vi "Test0823.vi"() -> ()   [LabVIEW 2016]
uses:
  LV-EDSDK-Distribution_0.2/Distribution/EDSDK-Labview.llb/EdsImageInfo.ctl
  LV-EDSDK-Distribution_0.2/Distribution/EDSDK-Labview.llb/kEdsProperties.ctl
  LV-EDSDK-Distribution_0.2/Distribution/EDSDK-Labview.llb/kEdsImageSrcs.ctl
  EDSDK131020CD(13.10.20)/EDSDK131020CD(13.10.20)/Windows/EDSDK_64/Dll/EDSDK.dll
  Dll for liveview/x64/Debug/Dll for liveview.dll
panel:
  out "2D Picture":picture
  out "Intensity Graph":u32[][](graph)
  out "output array":u32[][](array[numeric])
  out "return type 3":i32
  out "return type 2":i32
  in  "EdsRect":T1
  in  "EdsSize":cluster{"height":i32, "width":i32}
  out "return type":i32
  out "inStreamRef dup":i32
  out "outImageInfo":T2
  out "outDeviceInfo":T3
  out "error out":errorcluster
  in  "error in (no error)":errorcluster
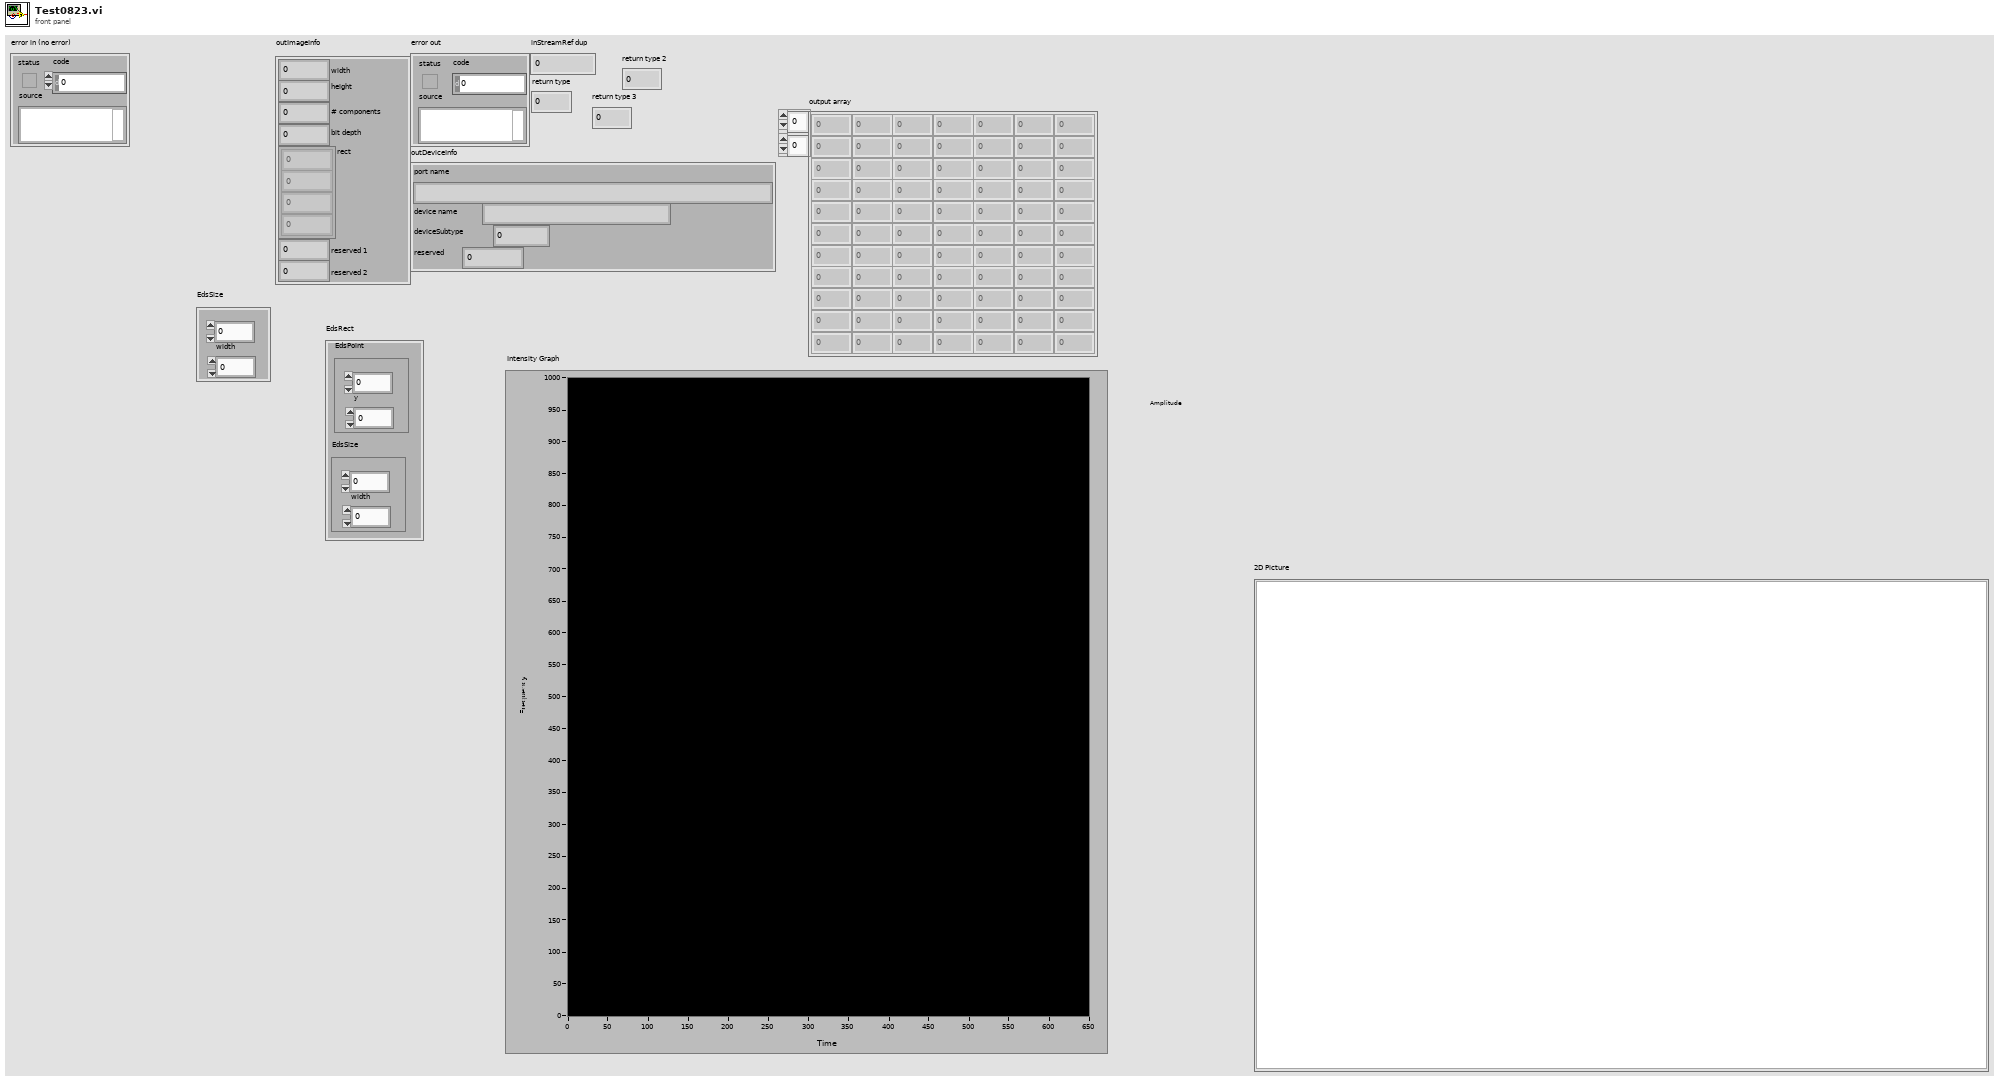
[diagram p1: front panel]
types:
  T1 = cluster{"EdsPoint":cluster{"x":i32, "y":i32}, "EdsSize":cluster{"height":i32, "width":i32}}
  T2 = typedef "EdsImageInfo.ctl" = cluster{"width":u32, "height":u32, "# components":u32, "bit depth":u32, "rect":u32[], "reserved 1":u32, "reserved 2":u32}
  T3 = cluster{"port name":string, "device name":string, "deviceSubtype":u32, "reserved":u32}
  T4 = typedef "kEdsProperties.ctl" = u32
  T5 = typedef "kEdsImageSrcs.ctl" = u32
  T6 = typedef "imagedata.ctl" = cluster{"image type":i32, "image depth":i32, "image":u8[], "mask":u8[], "colors":u32[], "Rectangle":cluster{"left":i16, "top":i16, "right":i16, "bottom":i16}}
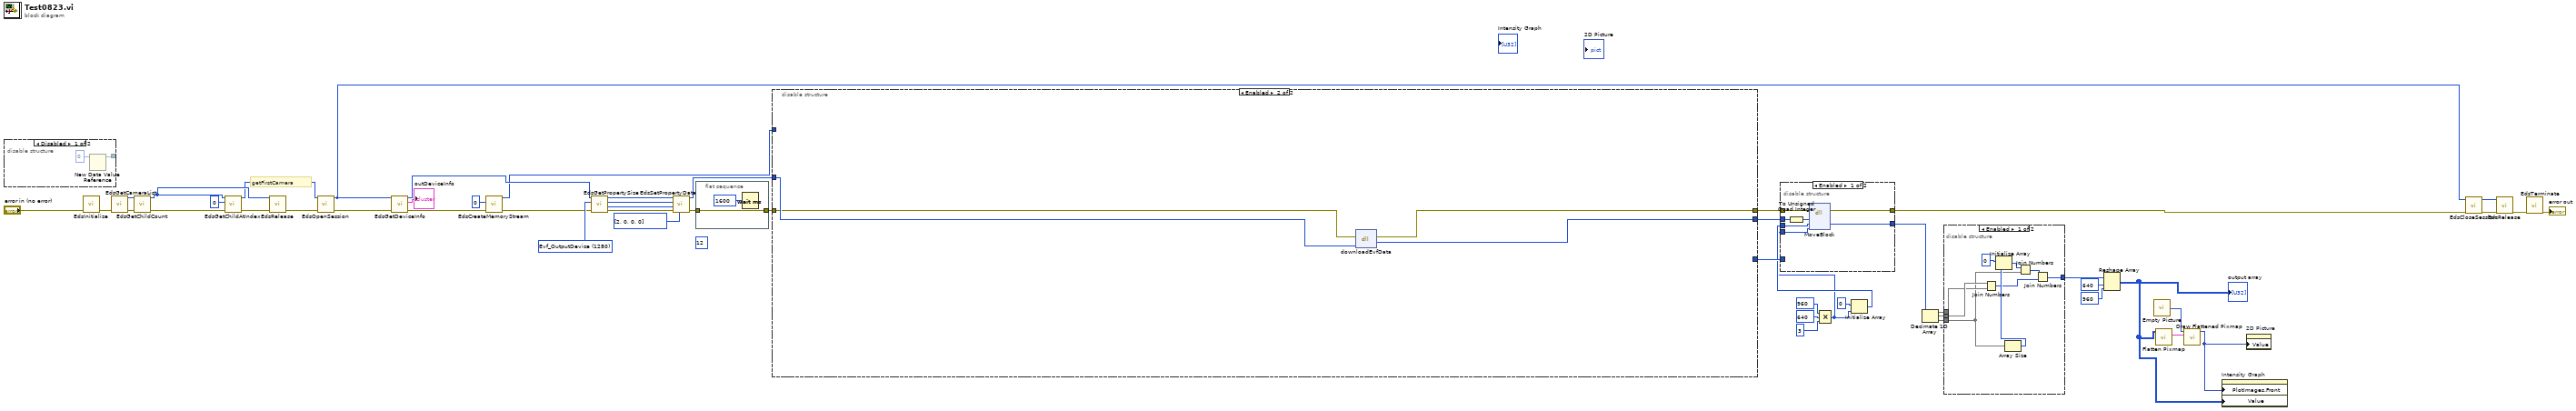
[diagram p0: block diagram]
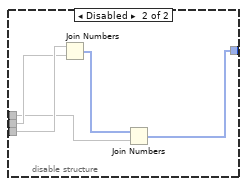
[diagram p2: hidden frame]
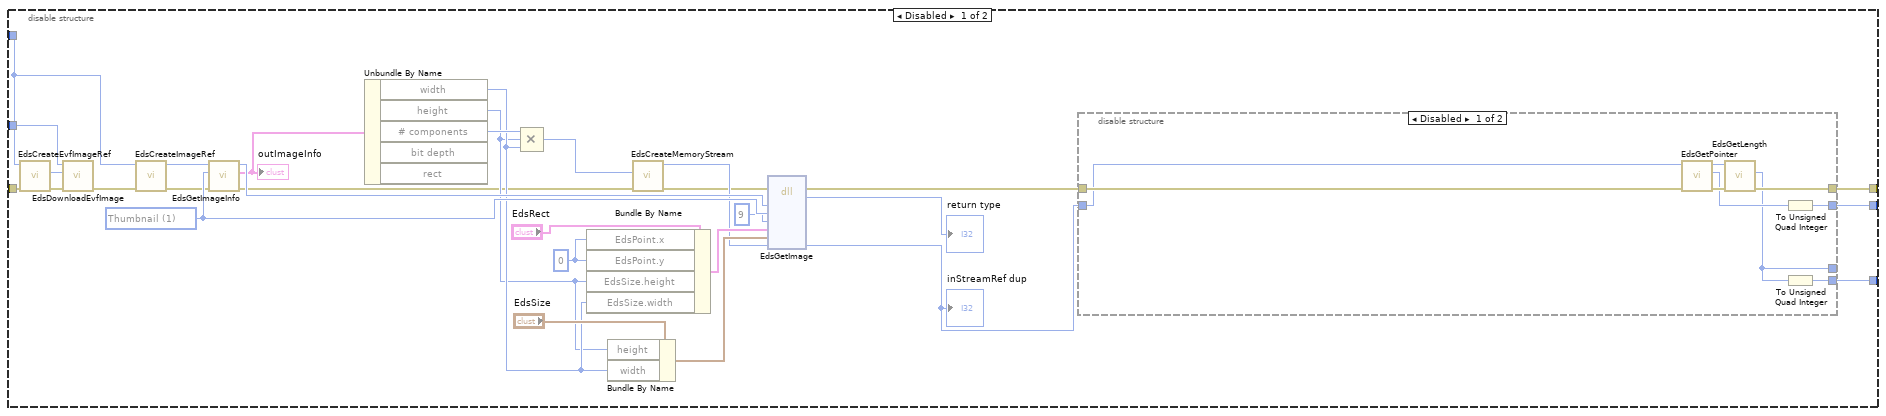
[diagram p3: hidden frame]
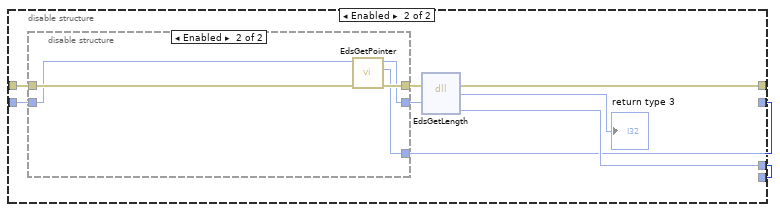
[diagram p4: hidden frame]
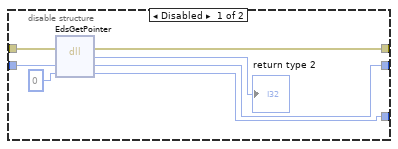
[diagram p5: hidden frame]
diagram:
  (unwired) u8 12 ("element")
  w36 = T4 1280 items=["Unknown"=65535, "ProductName"=2, "BodyID"=3, "OwnerName"=4, "MakerName"=5, "DateTime"=6, "FirmwareVersion"=7, "BatteryLevel"=8, "CFn"=9, "SaveTo"=11, "CurrentStorage"=12, "CurrentFolder"=13, "MyMenu"=14, "BatteryQuality"=16, "HDDirectoryStructure"=32, "ImageQuality"=256, "JpegQuality"=257, "Orientation"=258, "ICCProfile"=259, "FocusInfo"=260, "DigitalExposure"=261, "WhiteBalance"=262, "ColorTemperature"=263, "WhiteBalanceShift"=264, "Contrast"=265, "ColorSaturation"=266, "ColorTone"=267, "Sharpness"=268, "ColorSpace"=269, "ToneCurve"=270, "PhotoEffect"=271, "FilterEffect"=272, "ToningEffect"=273, "ParameterSet"=274, "ColorMatrix"=275, "PictureStyle"=276, "PictureStyleDesc"=277, "ETTL2Mode"=279, "PictureStyleCaption"=512, "Linear"=768, "ClickWBPoint"=769, "WBCoeffs"=770, "GPSVersionID"=2048, "GPSLatitudeRef"=2049, "GPSLatitude"=2050, "GPSLongitudeRef"=2051, "GPSLongitude"=2052, "GPSAltitudeRef"=2053, "GPSAltitude"=2054, "GPSTimeStamp"=2055, "GPSSatellites"=2056, "GPSStatus"=2057, "GPSMapDatum"=2066, "GPSDateStamp"=2077, "AtCapture_Flag"=2147483648, "AEMode"=1024, "DriveMode"=1025, "ISOSpeed"=1026, "MeteringMode"=1027, "AFMode"=1028, "Av"=1029, "Tv"=1030, "ExposureCompensation"=1031, "FlashCompensation"=1032, "FocalLength"=1033, "AvailableShots"=1034, "Bracket"=1035, "WhiteBalanceBracket"=1036, "LensName"=1037, "AEBracket"=1038, "FEBracket"=1039, "ISOBracket"=1040, "NoiseReduction"=1041, "FlashOn"=1042, "RedEye"=1043, "FlashMode"=1044, "LensStatus"=1046, "Artist"=1048, "Copyright"=1049, "DepthOfField"=1051, "EFCompensation"=1054, "Evf_OutputDevice"=1280, "Evf_Mode"=1281, "Evf_WhiteBalance"=1282, "Evf_ColorTemperature"=1283, "Evf_DepthOfFieldPreview"=1284, "Evf_Zoom"=1287, "Evf_ZoomPosition"=1288, "Evf_FocusAid"=1289, "Evf_Histogram"=1290, "Evf_ImagePosition"=1291, "Evf_HistogramStatus"=1292, "Evf_AFMode"=1294, "Evf_CoordinateSystem"=1344, "Evf_ZoomRect"=1345] ("inPropertyID")
  # "getFirstCamera"
  n1 = disable-structure shown="Disabled" {
    disable-tunnel: [w53 _] -> _
    frame Disabled {
      n2 = New Data Value Reference(data value=i64 0) -> (data value reference=w53:refnum<data-value>)  [unwired: 1 in, 1 out]
    }
    frame Enabled {
    }
  }
  n3 = call "EdsInitialize.vi"("error in (no error)"="error in (no error)") -> ("error out"=w51:errorcluster)  [unwired: 10 in]
  n4 = call "EdsGetCameraList.vi"("error in"=w51) -> ("error out"=w50:errorcluster, "outCameraListRef"=w46:u32)  [unwired: 9 in]
  n5 = call "EdsGetChildCount.vi"("error in"=w50, "inRef"=w46) -> ("error out"=w49:errorcluster, "inRef dup"=w45:u32)  [unwired: 7 in, 1 out]
  n6 = call "EdsGetChildAtIndex.vi"("error in"=w49, "index"=u32 0, "inRef"=w45) -> ("error out"=w47:errorcluster, "outRef"=w40:u32)  [unwired: 7 in]
  n7 = call "EdsRelease.vi"("error in"=w47, "inRef"=w45) -> ("error out"=w44:errorcluster)  [unwired: 7 in, 2 out]
  n8 = call "EdsOpenSession.vi"("error in"=w44, "inCameraRef"=w40) -> ("error out"=w38:errorcluster, "inCameraRef dup"=w39:u32)  [unwired: 8 in]
  n9 = call "EdsGetDeviceInfo.vi"("error in"=w38, "inCameraRef"=w39) -> ("error out"=w28:errorcluster, "outDeviceInfo"=→"outDeviceInfo":T3, "inCameraRef dup"=w29:u32)  [unwired: 7 in]
  n10 = call "EdsCreateMemoryStream.vi"("error in"=w28, "inBufferSize"=u32 0) -> ("error out"=w30:errorcluster, "outStreamRef"=w23:u32)  [unwired: 8 in]
  n11 = call "EdsGetPropertySize.vi"("error in"=w30, "inPropertyID"=w36, "inRef"=w29) -> ("error out"=w33:errorcluster, "outSize"=w32:u32, "inPropertyID dup"=w34:T4, "inRef dup"=w35:u32)  [unwired: 4 in, 1 out]
  n12 = call "EdsSetPropertyData.vi"("inPropertyData"=u8[] [2, 0, 0, 0], "error in"=w33, "inPropertySize"=w32, "inPropertyID"=w34, "inRef"=w35) -> ("error out"=w21:errorcluster, "inRef dup"=w26:u32)  [unwired: 5 in]
  n13 = flat-sequence {
    tunnel: w21 -> [w56]
    tunnel: [w56] -> w20
    frame #0 {
      n14 = Wait (ms)(milliseconds to wait=u32 1600) -> ()  [unwired: 1 out]
    }
  }
  n15 = disable-structure shown="Enabled" {
    disable-tunnel: w26 -> [w84 w119]
    disable-tunnel: [w72 _] -> w24
    disable-tunnel: w23 -> [w63 _]
    disable-tunnel: [w62 w117] -> w22
    disable-tunnel: w20 -> [w61 w118]
    disable-tunnel: [w60 w116] -> w6
    frame Disabled {
      w76 = 0 ("x")
      w81 = T5 1 items=["FullView", "Thumbnail", "Preview", "RAWThumbnail", "RAWFullView"] ("inImageSource")
      n16 = call "EdsCreateEvfImageRef.vi"("error in"=w61, "inStream"=w63) -> ("error out"=w86:errorcluster, "outEvfImage"=w85:u32)  [unwired: 7 in, 1 out]
      n17 = call "EdsDownloadEvfImage.vi"("error in"=w86, "inEvfImageRef"=w85, "inCameraRef"=w84) -> ("error out"=w66:errorcluster)  [unwired: 6 in, 2 out]
      n18 = call "EdsCreateImageRef.vi"("error in"=w66, "inStreamRef"=w63) -> ("error out"=w65:errorcluster, "outImageRef"=w64:u32)  [unwired: 8 in]
      n19 = call "EdsGetImageInfo.vi"("error in"=w65, "inImageSource"=w81, "inImageRef"=w64) -> ("error out"=w58:errorcluster, "outImageInfo"=w82:T2, "inImageRef dup"=w83:u32)  [unwired: 6 in]
      "outImageInfo" <- w82
      n20 = Unbundle By Name(w82) -> ("width"=w71:u32, "height"=w70:u32, "# components"=w80:u32)  [unwired: 2 out]
      n21 = Compound Arithmetic op=MULTIPLY(w80, w70, w71) -> (w68:u32)
      n22 = Bundle By Name(cluster="EdsRect", "EdsPoint.x"=w76, "EdsPoint.y"=w76, "EdsSize.height"=w70, "EdsSize.width"=w71) -> (w74:T1)
      n23 = Bundle By Name(cluster="EdsSize", "height"=w70, "width"=w71) -> (w73:cluster{"height":i32, "width":i32})
      n24 = call "EdsCreateMemoryStream.vi"("error in"=w58, "inBufferSize"=w68) -> ("error out"=w57:errorcluster, "outStreamRef"=w67:u32)  [unwired: 8 in]
      n25 = dll-call lib="D:/All Users/Summer2019/Camera_po_sheng/Canon/EDSDK131020CD(13.10.20)/EDSDK131020CD(13.10.20)/Windows/EDSDK_64/Dll/EDSDK.dll" fn="EdsGetImage"(error in=w57, "inImageRef"=w83, "inImageSource"=w81, "inImageType"=9, "inSrcRect"=w74, "inDstSize"=w73, "outStreamRef"=w67) -> (error out=w59:errorcluster, "return type"=→"return type":i32, "outStreamRef"=w69:u32)  [unwired: 7 in, 1 out]
      "inStreamRef dup" <- w69
      n26 = disable-structure shown="Disabled" {
        disable-tunnel: w59 -> [w92 w103]
        disable-tunnel: [w91 w97] -> w72
        disable-tunnel: w69 -> [w90 w102]
        disable-tunnel: [w89 w98] -> w62
        disable-tunnel: [w88 w96] -> w60
        disable-tunnel: [w87 w97] -> _
        frame Disabled {
          n27 = call "EdsGetPointer.vi"("error in"=w92, "inStream"=w90) -> ("error out"=w95:errorcluster, "outPointer"=w93:u32, "inStream dup"=w94:u32)  [unwired: 7 in]
          n28 = call "EdsGetLength.vi"("error in"=w95, "inStreamRef"=w94) -> ("error out"=w89:errorcluster, "outLength"=w87:u32)  [unwired: 7 in, 1 out]
          n29 = To Unsigned Quad Integer(1:w93) -> (0:w88:u64)
          n30 = To Unsigned Quad Integer(1:w87) -> (0:w91:u64)
        }
        frame Enabled {
          n31 = disable-structure shown="Enabled" {
            disable-tunnel: w103 -> [w110 w115]
            disable-tunnel: w102 -> [w109 w113]
            disable-tunnel: [w108 w111] -> w101
            disable-tunnel: [w106 w114] -> w99
            disable-tunnel: [w105 w112] -> w96
            frame Disabled {
              n32 = dll-call lib="D:/All Users/Summer2019/Camera_po_sheng/Canon/EDSDK131020CD(13.10.20)/EDSDK131020CD(13.10.20)/Windows/EDSDK_64/Dll/EDSDK.dll" fn="EdsGetPointer"(error in=w110, "inStreamRef"=w109, "outPointer"=i64 0) -> (error out=w106:errorcluster, "return type"=→"return type 2":i32, "inStreamRef"=w108:i32, "outPointer"=w105:i64)  [unwired: 2 in, 1 out]
            }
            frame Enabled {
              n33 = call "EdsGetPointer.vi"("error in"=w115, "inStream"=w113) -> ("error out"=w114:errorcluster, "outPointer"=w112:u32, "inStream dup"=w111:u32)  [unwired: 7 in]
            }
          }
          n34 = dll-call lib="D:/All Users/Summer2019/Camera_po_sheng/Canon/EDSDK131020CD(13.10.20)/EDSDK131020CD(13.10.20)/Windows/EDSDK_64/Dll/EDSDK.dll" fn="EdsGetLength"(error in=w99, "inStreamRef"=w101) -> (error out=w98:errorcluster, "return type"=→"return type 3":i32, "ouLength"=w97:u32)  [unwired: 4 in, 1 out]
        }
      }
    }
    frame Enabled {
      n35 = dll-call lib="D:/All Users/Summer2019/Camera_po_sheng/Dll for liveview/x64/Debug/Dll for liveview.dll" fn="downloadEvfData"(error in=w118, "CamRef"=w119) -> (error out=w117:errorcluster, "return type"=w116:i64)  [unwired: 3 in, 1 out]
    }
  }
  n36 = Compound Arithmetic op=MULTIPLY(960 ("dimension size"), 640 ("dimension size"), 3 ("dimension size")) -> (w14:i32)
  n37 = Initialize Array ("初始化数组")(u8 0 ("element"), w14) -> (w15:u8[])
  n38 = disable-structure shown="Enabled" {
    disable-tunnel: [w126 w127] -> w4
    disable-tunnel: w6 -> [w125 _]
    disable-tunnel: w22 -> [w124 w127]
    disable-tunnel: w24 -> [_ _]
    disable-tunnel: w15 -> [w123 _]
    disable-tunnel: w14 -> [w122 _]
    disable-tunnel: [w120 _] -> w7
    frame Enabled {
      n39 = To Unsigned Quad Integer(1:w125) -> (0:w121:u64)
      n40 = dll-call lib="LabVIEW" fn="MoveBlock"(error in=w124, "src"=w121, "dst"=w123, "size"=w122) -> (error out=w126:errorcluster, "dst"=w120:u8[])  [unwired: 5 in, 1 out]
    }
    frame Disabled {
    }
  }
  n41 = Decimate 1D Array(w7) -> (w12:u8[], w13:u8[], w11:u8[])
  n42 = disable-structure shown="Enabled" {
    disable-tunnel: w13 -> [w136 w138]
    disable-tunnel: w12 -> [w135 w137]
    disable-tunnel: w11 -> [w131 w139]
    disable-tunnel: [w128 w140] -> w10
    frame Enabled {
      n43 = Join Numbers(hi=w136, lo=w135) -> ((hi.lo)=w129:u16[])
      n44 = Array Size(array=w131) -> (size(s)=w133:i32)
      n45 = Initialize Array(u8 0, w133) -> (w132:u8[])
      n46 = Join Numbers(hi=w132, lo=w131) -> ((hi.lo)=w130:u16[])
      n47 = Join Numbers(hi=w130, lo=w129) -> ((hi.lo)=w128:u32[])
    }
    frame Disabled {
      n48 = Join Numbers(hi=w139, lo=w138) -> ((hi.lo)=w141:u16[])
      n49 = Join Numbers(hi=w141, lo=w137) -> ((hi.lo)=w140:u32[])
    }
  }
  n50 = Reshape Array(w10, 640 ("dimension size"), 960 ("dimension size")) -> (w1:u32[][])
  "output array" <- w1
  n51 = call "Empty Picture"() -> ("empty picture"=w2:picture)
  n52 = call <vilib>:"Flatten Pixmap.vi"("24-bit pixmap"=w1) -> ("image data"=w5:T6)  [unwired: 10 in]
  n53 = call <vilib>:"Draw Flattened Pixmap.vi"("image data"=w5, "picture"=w2) -> ("new picture"=w3:picture)  [unwired: 7 in]
  n54 = property on="Intensity Graph" class="IntGraph (strict)"("PlotImages.Front"=w3, "Value"=w1) -> ()  [unwired: 2 in, 2 out]
  n55 = property on="2D Picture" class="Pict"("Value"=w3) -> ()  [unwired: 2 in, 2 out]
  n56 = call "EdsCloseSession.vi"("error in"=w4, "inCameraRef"=w39) -> ("error out"=w25:errorcluster, "inCameraRef dup"=w43:u32)  [unwired: 8 in]
  n57 = call "EdsRelease.vi"("error in"=w25, "inRef"=w43) -> ("error out"=w42:errorcluster)  [unwired: 7 in, 2 out]
  n58 = call "EdsTerminate.vi"("error in"=w42) -> ("error out"=→"error out":errorcluster)  [unwired: 10 in]
